vi "DC Attenuation Pre-Processing.vi"(6 "Username (\"\")":string, 7 "Fields In":T1[](array[typedef]), 8 "error in (no error)":errorcluster, 10 "Test Configuration (\"\")":string, 11 "Test_ID (\"\")":string) -> (0 "error out":errorcluster, 1 "Files Found?":bool, 2 "New Test Configuration":string, 3 "Dup Test_ID":string, 5 "Fields Out":T1[](array[typedef]))   [LabVIEW 2011]
uses:
  server/database/Fields/Field Record.ctl
  server/database/Fields/Field DataTypes.ctl
  server/database/Fields/Field NextItem.ctl
  TypeDefs/DCA Limit.ctl
  TypeDefs/DCA Limit Quantity.ctl
  TypeDefs/DCA Limit Comparison.ctl
  TypeDefs/DCA Limit Operation.ctl
  Test Referential Limit.ctl
  server/database/Fields/Field System Fields.ctl
  LIB/DC Attenuation Version.vi
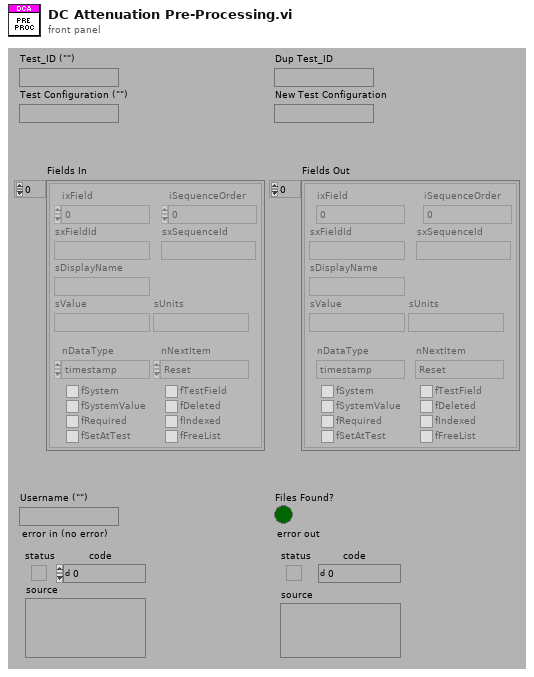
[diagram p1: front panel]
types:
  T1 = typedef "Field Record.ctl" = cluster{"ixField":i32, "iSequenceOrder":i32, "sxFieldId":string, "sxSequenceId":string, "sDisplayName":string, "sValue":string, "sUnits":string, "nDataType":T2, "nNextItem":T3, "fSystem":bool, "fSystemValue":bool, "fRequired":bool, "fSetAtTest":bool, "fTestField":bool, "fDeleted":bool, "fIndexed":bool, "fFreeList":bool}
  T2 = typedef "Field DataTypes.ctl" = enum32{"text", "numeric", "list", "timestamp", "boolean"}
  T3 = typedef "Field NextItem.ctl" = enum32{"Reset", "Retain", "Auto-Increment"}
  T4 = cluster{"Ref Limit":bool, "Ref Type":bool, "Model":bool, "Serial":bool, "Run Type":bool, "Run":bool, "Field":bool, "Field Value":bool}
  T5 = typedef "Field System Fields.ctl" = enum32{"Company", "End_Timestamp", "Model_Number", "Operator", "Serial_Number", "Start_Timestamp", "Step_Number", "Step_Tag", "Test_Run", "Test_Sequence", "Test_Station", "Test_Station_Name", "Test_Status", "Test_Type", "Test_Version", "Spartan_Version_Created", "Spartan_Version_Current"}
  T6 = typedef "DCA Limit.ctl" = cluster{"Parameter":T7, "Comparison":T8, "Operation":T9, "Value":dbl, "Referential Limit":T10}
  T7 = typedef "DCA Limit Quantity.ctl" = enum16{"Attenuation", "Zin", "Zout", "R1", "R2", "R3", "Rab", "Rac", "Rbc"}
  T8 = typedef "DCA Limit Comparison.ctl" = enum16{">", ">=", "<", "<="}
  T9 = typedef "DCA Limit Operation.ctl" = enum16{"+", "-"}
  T10 = typedef "Test Referential Limit.ctl" = cluster{"Ref Limit":bool, "Ref Type":enum16{"Current", "Specify"}, "Model":string, "Serial":string, "Run Type":enum16{"Most Recent", "Run #", "Match Field"}, "Run":i32, "Field":string, "Field Value":string}
  T11 = typedef "DCA Test Parameters.ctl" = cluster{"Stimulus":T12, "Measurement":T13, "Limits":T6[], "Normalization":T16}
  T12 = typedef "DCA Stimulus Parameters.ctl" = cluster{"Use Instrument":bool, "Normalize":bool, "Blank Screen":bool, "Measurement Type":enum16{"Voltage DC", "Voltage DC Ratio", "Voltage AC", "Current DC", "Current AC", "Resistance", "Fresistance", "Frequency", "Period", "Continuity", "Diode"}, "Range":enum16{"Auto", "Minimum", "Maximum", "100", "1,000", "10,000", "100,000", "1,000,000", "10,000,000", "100,000,000"}, "Resolution":enum16{"Auto", "4 1/2", "5 1/2", "6 1/2"}}
  T13 = typedef "DCA Measurement Cluster.ctl" = cluster{"Topology":T14, "Lock Topology":bool, "ATTN Calc":T15, "Zo":dbl}
  T14 = typedef "DCA Topology.ctl" = enum32{"PI-Network", "T-Network"}
  T15 = typedef "DCA Attenuation Calculation.ctl" = enum32{"Power", "Voltage"}
  T16 = typedef "DCA Calibration State.ctl" = cluster{"Normalized?":bool, "Rab Value":dbl, "Rac Value":dbl, "Rbc Value":dbl}
  T17 = cluster{"Parameter":bool, "Comparison":bool, "Operation":bool, "Value":bool, "Referential Limit":cluster{"Ref Limit":bool, "Ref Type":bool, "Model":bool, "Serial":bool, "Run Type":bool, "Run":bool, "Field":bool, "Field Value":bool}}
  T18 = typedef "Connection Refnum.ctl" = cluster{"Environment Handle":i32, "Connection Handle":i32}
  T19 = typedef "TDMS File.ctl" = cluster{"File Path":path, "Run Data":T20[], "Serial Number":string, "Model Number":string, "Test Type":string}
  T20 = typedef "TDMS Run.ctl" = cluster{"Channel Data":T21[], "Custom Fields":T1[], "Run ID":string}
  T21 = typedef "TDMS Channel (Sxx).ctl" = cluster{"Channel Name":string, "Waveform":dbl[], "Unit":string, "List value":string}
  T22 = typedef "OGAB Version.ctl" = cluster{"Version":string, "Build Number":u32, "Build Date/Time":dbl}
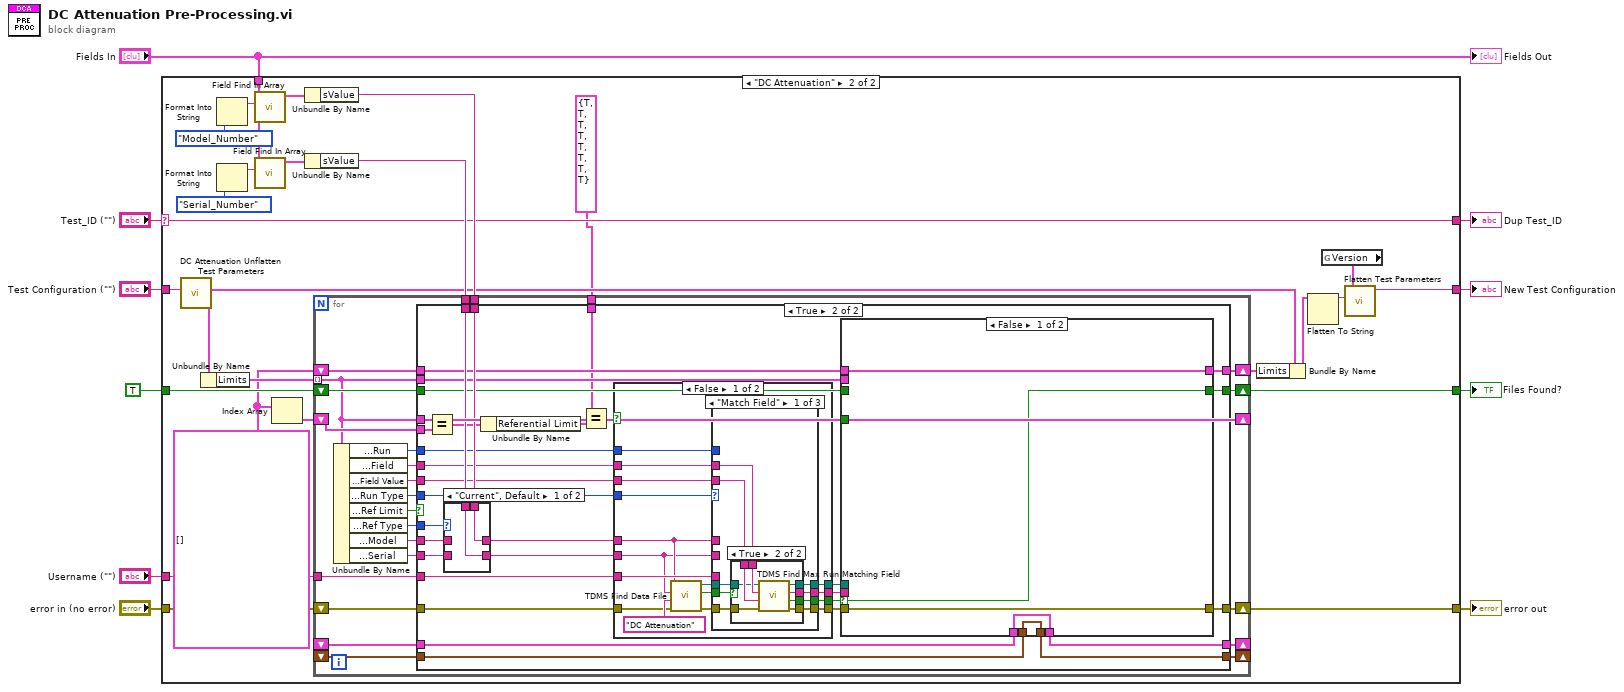
[diagram p0: block diagram]
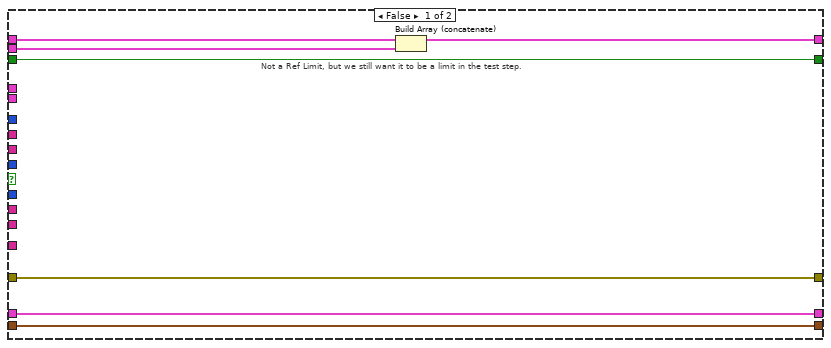
[diagram p3: hidden frame]
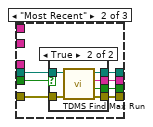
[diagram p5: hidden frame]
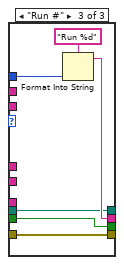
[diagram p7: hidden frame]
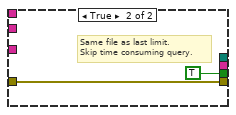
[diagram p8: hidden frame]
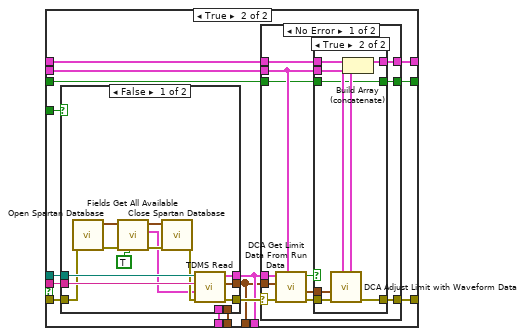
[diagram p9: hidden frame]
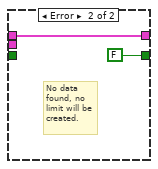
[diagram p12: hidden frame]
diagram:
  n1 = case shown="\"DC Attenuation\"" "Test_ID (\"\")" {
    selector: "Test_ID (\"\")" -> [w12 w20]
    tunnel: [w12 w20] -> w10
    tunnel: "Test Configuration (\"\")" -> [w14 w40]
    tunnel: [w14 w36] -> w8
    tunnel: "error in (no error)" -> [w13 w35]
    tunnel: [w13 w34] -> w4
    tunnel: "Fields In" -> [_ w27]
    tunnel: "Username (\"\")" -> [_ w24]
    tunnel: TRUE -> [w11 w19]
    tunnel: [w11 w18] -> w1
    frame Default {
    }
    frame "DC Attenuation" {
      w17 = T6[] [] ("Limits")
      n2 = call "DC Attenuation Unflatten Test Parameters.vi"("Parameter String"=w40) -> ("DC Attenuation Test Parameters"=w23:T11)  [unwired: 1 in, 9 out]
      n3 = Unbundle By Name(w23) -> ("Limits"=w22:T6[])
      n4 = Format Into String(Field_System_Fields."Model_Number" ("System Field to Replace (Serial Number)")) -> (resulting string=w31:string)  [unwired: 3 in, 1 out]
      n5 = Format Into String(Field_System_Fields."Serial_Number" ("System Field to Replace (Serial Number)")) -> (resulting string=w30:string)  [unwired: 3 in, 1 out]
      n6 = call "Field Find In Array.vi"("FieldID or Display Name(\"\")"=w31, "Field Array"=w27) -> ("Field"=w33:T1)  [unwired: 1 in, 8 out]
      n7 = call "Field Find In Array.vi"("FieldID or Display Name(\"\")"=w30, "Field Array"=w27) -> ("Field"=w28:T1)  [unwired: 1 in, 8 out]
      n8 = Index Array(array=w17) -> (element=w16:T6)  [unwired: 1 in]
      n9 = Unbundle By Name(w33) -> ("sValue"=w26:string)
      n10 = Unbundle By Name(w28) -> ("sValue"=w25:string)
      n11 = for {
        tunnel: w22 -> [w46] mode=indexing
        shift-right: [w57] -> w34
        shift-left: w35 -> [w58]
        tunnel: w26 -> [w56]
        tunnel: w25 -> [w55]
        tunnel: w24 -> [w52]
        shift-right: [w50] -> w21
        shift-left: w17 -> [w51]
        shift-right: [w48] -> w18
        shift-left: w19 -> [w49]
        shift-right: [w46] -> _
        shift-left: w16 -> [w47]
        tunnel: T4 {"Ref Limit"=TRUE, "Ref Type"=TRUE, "Model"=TRUE, "Serial"=TRUE, "Run Type"=TRUE, "Run"=TRUE, "Field"=TRUE, "Field Value"=TRUE} ("Referential Limit") -> [w45]
        shift-right: [w44] -> _
        shift-left: _ -> [w42]
        shift-right: [w43] -> _
        shift-left: _ -> [w41]
        n12 = Unbundle By Name(w46) -> ("Referential Limit.Run"=w53:i32, "Referential Limit.Field"=w59:string, "Referential Limit.Field Value"=w60:string, "Referential Limit.Run Type"=w61:enum16{"Most Recent", "Run #", "Match Field"}, "Referential Limit.Ref Limit"=w54:bool, "Referential Limit.Ref Type"=w62:enum16{"Current", "Specify"}, "Referential Limit.Model"=w63:string, "Referential Limit.Serial"=w64:string)
        n13 = case shown="True" w54 {
          tunnel: w46 -> [w69 w92]
          tunnel: w64 -> [_ w102]
          tunnel: w63 -> [_ w103]
          tunnel: w62 -> [_ w104]
          tunnel: w61 -> [_ w99]
          tunnel: w60 -> [_ w98]
          tunnel: w59 -> [_ w97]
          tunnel: w58 -> [w71 w84]
          tunnel: [w71 w91] -> w57
          tunnel: w56 -> [_ w101]
          tunnel: w55 -> [_ w100]
          tunnel: w53 -> [_ w93]
          tunnel: w52 -> [_ w90]
          tunnel: w51 -> [w70 w89]
          tunnel: [w68 w88] -> w50
          tunnel: w49 -> [w67 w87]
          tunnel: [w67 w86] -> w48
          tunnel: w47 -> [_ w81]
          tunnel: w46 -> [_ w82]
          tunnel: w45 -> [_ w80]
          tunnel: [w66 w78] -> w44
          tunnel: [w65 w77] -> w43
          tunnel: w42 -> [w66 w76]
          tunnel: w41 -> [w65 w75]
          frame False {
            # "Not a Ref Limit, but we still want it to be a limit in the test step."
            n14 = Build Array (concatenate)(w70, w69) -> (w68:T6[])
          }
          frame True {
            n15 = Equal?(x=w82, y=w81) -> (x = y?=w74:T17)
            n16 = case shown="\"Current\", Default" w104 {
              tunnel: w103 -> [_ w229]
              tunnel: w102 -> [_ w228]
              tunnel: [w227 w229] -> w96
              tunnel: [w226 w228] -> w95
              tunnel: w101 -> [w227 _]
              tunnel: w100 -> [w226 _]
              frame "Current", Default {
              }
              frame "Specify" {
              }
            }
            n17 = Unbundle By Name(w74) -> ("Referential Limit"=w73:T4)
            n18 = Equal?(x=w80, y=w73) -> (x = y?=w79:bool)
            n19 = case shown="False" w79 {
              tunnel: w99 -> [w120 _]
              tunnel: w98 -> [w119 _]
              tunnel: w97 -> [w118 _]
              tunnel: w96 -> [w108 _]
              tunnel: w95 -> [w107 _]
              tunnel: [w117 _] -> w94
              tunnel: w93 -> [w116 _]
              tunnel: w90 -> [w115 _]
              tunnel: [w114 w164] -> w85
              tunnel: w84 -> [w110 w164]
              tunnel: [w113 _] -> w83
              tunnel: [w112 TRUE ("Found?")] -> w72
              frame False {
                n20 = call "TDMS Find Data File.vi"("error in (no error)"=w110, "Test Type"="DC Attenuation" ("Value"), "Serial Number"=w107, "Model Number"=w108) -> ("error out"=w109:errorcluster, "Found?"=w105:bool, "TDMS Path"=w106:path)  [unwired: 5 in]
                n21 = case shown="\"Match Field\"" w120 {
                  tunnel: w118 -> [w129 _ _]
                  tunnel: w119 -> [w128 _ _]
                  tunnel: w109 -> [w123 w143 w158]
                  tunnel: [w127 w147 w158] -> w114
                  tunnel: w108 -> [_ _ _]
                  tunnel: w107 -> [_ _ _]
                  tunnel: [w126 w146 w159] -> w113
                  tunnel: [w125 w145 w160] -> w117
                  tunnel: w116 -> [_ _ w161]
                  tunnel: w115 -> [_ _ _]
                  tunnel: [w124 w144 w157] -> w112
                  tunnel: w106 -> [w122 w142 w159]
                  tunnel: w105 -> [w121 w141 w157]
                  frame "Match Field" {
                    n22 = case shown="True" w121 {
                      selector: w121 -> [w130 _]
                      tunnel: w129 -> [_ w140]
                      tunnel: w128 -> [_ w139]
                      tunnel: w122 -> [w132 w138]
                      tunnel: w123 -> [w131 w137]
                      tunnel: [w131 w136] -> w127
                      tunnel: [w132 w135] -> w126
                      tunnel: [_ w134] -> w125
                      tunnel: [w130 w133] -> w124
                      frame False {
                      }
                      frame True {
                        n23 = call "TDMS Find Max Run Matching Field.vi"("error in (no error)"=w137, "Property Value"=w139, "Property Name"=w140, "TDMS File Path"=w138) -> ("error out"=w136:errorcluster, "Found?"=w133:bool, "Run ID"=w134:string, "TDMS File Path Out"=w135:path)  [unwired: 4 in]
                      }
                    }
                  }
                  frame "Most Recent" {
                    n24 = case shown="True" w141 {
                      selector: w141 -> [w148 _]
                      tunnel: w142 -> [w150 w156]
                      tunnel: w143 -> [w149 w155]
                      tunnel: [w149 w154] -> w147
                      tunnel: [w150 w153] -> w146
                      tunnel: [_ w152] -> w145
                      tunnel: [w148 w151] -> w144
                      frame False {
                      }
                      frame True {
                        n25 = call "TDMS Find Max Run.vi"("error in (no error)"=w155, "TDMS File Path"=w156) -> ("error out"=w154:errorcluster, "Found?"=w151:bool, "Run ID"=w152:string, "TDMS File Path Out"=w153:path)  [unwired: 6 in]
                      }
                    }
                  }
                  frame "Run #" {
                    n26 = Format Into String(format string="Run %d", w161) -> (resulting string=w160:string)  [unwired: 2 in, 1 out]
                  }
                }
              }
              frame True {
                # "Same file as last limit.\nSkip time consuming query."
              }
            }
            n27 = case shown="False" w72 {
              selector: w72 -> [w165 _]
              tunnel: w83 -> [_ w184]
              tunnel: w94 -> [_ w183]
              tunnel: w92 -> [_ w181]
              tunnel: [w168 w180] -> w91
              tunnel: w89 -> [w169 w179]
              tunnel: [w169 w178] -> w88
              tunnel: w87 -> [_ w177]
              tunnel: [w165 w176] -> w86
              tunnel: w85 -> [w168 w175]
              tunnel: w79 -> [_ w174]
              tunnel: [w166 w173] -> w78
              tunnel: [w167 w172] -> w77
              tunnel: w76 -> [w166 w171]
              tunnel: w75 -> [w167 w170]
              frame False {
              }
              frame True {
                n28 = case shown="False" w174 {
                  tunnel: w184 -> [w197 _]
                  tunnel: w183 -> [w196 _]
                  tunnel: [w195 w200] -> w182
                  tunnel: [w194 w198] -> w172
                  tunnel: [w193 w199] -> w173
                  tunnel: w175 -> [w187 w200]
                  tunnel: w171 -> [_ w199]
                  tunnel: w170 -> [_ w198]
                  frame False {
                    n29 = call "Open Spartan Database.vi"("error in (no error)"=w187) -> ("error out"=w188:errorcluster, "Connection Refnum"=w189:T18)  [unwired: 9 in]
                    n30 = call "Fields Get All Available.vi"("Combine All? (f)"=TRUE, "error in (no error)"=w188, "Connection Refnum"=w189) -> ("error out"=w191:errorcluster, "System or ALL Combined Fields"=w185:T1[], "Connection Refnum"=w192:T18)  [unwired: 3 in, 3 out]
                    n31 = call "Close Spartan Database.vi"("error in (no error)"=w191, "Connection Refnum"=w192) -> ("error out"=w186:errorcluster)  [unwired: 9 in]
                    n32 = call "TDMS Read.vi"("error in (no error)"=w186, "System or ALL Combined Fields"=w185, "Run String"=w196, "TDM File Path"=w197) -> ("error out"=w195:errorcluster, "Run Waveforms"=w194:waveform(dbl)[], "File Information"=w193:T19)  [unwired: 3 in, 2 out]
                  }
                  frame True {
                    # "Same file as last limit.\nSkip time consuming read."
                  }
                }
                n33 = case shown="No Error" w182 {
                  selector: w182 -> [w212 _]
                  tunnel: w181 -> [w206 _]
                  tunnel: [w207 _] -> w180
                  tunnel: w172 -> [w210 _]
                  tunnel: w173 -> [w211 _]
                  tunnel: w179 -> [w204 w225]
                  tunnel: [w203 w225] -> w178
                  tunnel: w177 -> [w202 _]
                  tunnel: [w201 FALSE] -> w176
                  frame No Error {
                    n34 = call "DCA Get Limit Data From Run Data.vi"("Limit"=w206, "error in (no error)"=w212, "Run Waveforms"=w210, "File Information"=w211) -> ("error out"=w209:errorcluster, "Data Waveform"=w205:waveform(dbl), "Found?"=w208:bool)  [unwired: 5 out]
                    n35 = case shown="True" w208 {
                      selector: w208 -> [w213 _]
                      tunnel: w209 -> [w215 w223]
                      tunnel: [w215 w222] -> w207
                      tunnel: w206 -> [_ w221]
                      tunnel: w205 -> [_ w220]
                      tunnel: w204 -> [w214 w219]
                      tunnel: [w214 w217] -> w203
                      tunnel: w202 -> [_ w216]
                      tunnel: [w213 w216] -> w201
                      frame False {
                        # "No data\nfound, no\nlimit will be\ncreated."
                      }
                      frame True {
                        n36 = call "DCA Adjust Limit with Waveform Data.vi"("Limit"=w221, "error in (no error)"=w223, "Data Waveform"=w220) -> ("error out"=w222:errorcluster, "Modified Limit"=w218:T6)  [unwired: 7 out]
                        n37 = Build Array (concatenate)(w219, w218) -> (w217:T6[])
                      }
                    }
                  }
                  frame Error {
                    # "No data\nfound, no\nlimit will be\ncreated."
                  }
                }
              }
            }
          }
        }
      }
      n38 = Bundle By Name(cluster=w23, "Limits"=w21) -> (w37:T11)
      n39 = Flatten To String(anything=w37) -> (data string=w39:string)  [unwired: 1 in, 4 out]
      n40 = global read "DC Attenuation Version.vi" "Version"() -> (w38:T22)
      n41 = call "Flatten Test Parameters.vi"("Flattened Test Parameters (\"\")"=w39, "Test Version"=w38) -> ("Flattened Test Parameters with Version"=w36:string)  [unwired: 1 in, 4 out]
    }
  }
  "error out" <- w4
  "New Test Configuration" <- w8
  "Dup Test_ID" <- w10
  "Files Found?" <- w1
  "Fields Out" <- "Fields In"
